vi "Coff creator.vi"(11 "notes":i32) -> (2 "Array":i32[](array[numeric]), 3 "Array 2":dbl[](array[numeric]))   [LabVIEW 2025]
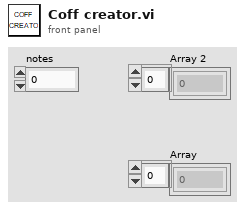
[diagram p1: front panel]
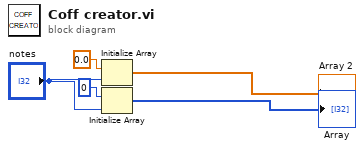
[diagram p0: block diagram]
diagram:
  n1 = Initialize Array(0.0 ("velocity"), "notes") -> (→"Array 2":dbl[])
  n2 = Initialize Array(0 ("style"), "notes") -> (→"Array":i32[])
